vi "clfnandsubvi.vi"   [LabVIEW 2014]
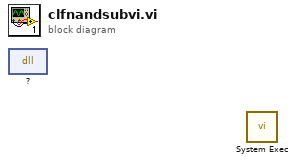
[diagram p0: block diagram]
diagram:
  n1 = dll-call lib="?" fn="?"() -> ()  [unwired: 4 in, 2 out]
  n2 = call <vilib>:"System Exec.vi"() -> ()  [unwired: 8 in, 4 out]
